vi "测试类型3can请求.vi"(3 "输入切换ID":u8, 4 "输出切换ID":u8) -> (1 "发送成功?":bool)   [LabVIEW 2010]
panel:
  in  "DataLen":i16
  in  "Data":u8[](array[numeric])
  in  "CANPort":u16
  in  "Synchronization":i32(ring)=1 items=["Synchronization"=1, "Asynchronization"=0]
  in  "WriteTimeOut":u32=5000 caption="ms"
  in  "Baudrate":u32(ring)=1000 caption="K" items=["10"=10, "20"=20, "50"=50, "100"=100, "125"=125, "250"=250, "500"=500, "800"=800, "1000"=1000]
  in  "Send_MSG":T1(array[cluster])=[{"Flags"=4, "ID(HEX)"=0, "Data "=[0, 0, 0, 0, 0, 0, 0, 0]}, {"Flags"=4, "ID(HEX)"=0, "Data "=[0, 0, 0, 0, 0, 0, 0, 1]}, {"Flags"=4, "ID(HEX)"=0, "Data "=[0, 0, 0, 0, 0, 0, 0, 2]}, {"Flags"=4, "ID(HEX)"=0, "Data "=[0, 0, 0, 0, 0, 0, 0, 3]}, {"Flags"=4, "ID(HEX)"=0, "Data "=[0, 0, 0, 0, 0, 0, 0, 4]}, {"Flags"=4, "ID(HEX)"=0, "Data "=[0, 0, 0, 0, 0, 0, 0, 5]}, {"Flags"=4, "ID(HEX)"=0, "Data "=[0, 0, 0, 0, 0, 0, 0, 6]}, {"Flags"=4, "ID(HEX)"=0, "Data "=[0, 0, 0, 0, 0, 0, 0, 7]}, {"Flags"=4, "ID(HEX)"=0, "Data "=[0, 0, 0, 0, 0, 0, 0, 8]}, {"Flags"=4, "ID(HEX)"=0, "Data "=[0, 0, 0, 0, 0, 0, 0, 9]}, {"Flags"=4, "ID(HEX)"=0, "Data "=[0, 0, 0, 0, 0, 0, 1, 0]}, {"Flags"=4, "ID(HEX)"=0, "Data "=[0, 0, 0, 0, 0, 0, 1, 1]}, {"Flags"=4, "ID(HEX)"=0, "Data "=[0, 0, 0, 0, 0, 0, 1, 2]}, {"Flags"=4, "ID(HEX)"=0, "Data "=[0, 0, 0, 0, 0, 0, 1, 3]}, {"Flags"=4, "ID(HEX)"=0, "Data "=[0, 0, 0, 0, 0, 0, 1, 4]}, {"Flags"=4, "ID(HEX)"=0, "Data "=[0, 0, 0, 0, 0, 0, 1, 5]}, {"Flags"=4, "ID(HEX)"=0, "Data "=[0, 0, 0, 0, 0, 0, 1, 6]}, {"Flags"=4, "ID(HEX)"=0, "Data "=[0, 0, 0, 0, 0, 0, 1, 7]}, {"Flags"=4, "ID(HEX)"=0, "Data "=[0, 0, 0, 0, 0, 0, 1, 8]}, {"Flags"=4, "ID(HEX)"=0, "Data "=[0, 0, 0, 0, 0, 0, 1, 9]}, {"Flags"=4, "ID(HEX)"=0, "Data "=[0, 0, 0, 0, 0, 0, 2, 0]}, {"Flags"=4, "ID(HEX)"=0, "Data "=[0, 0, 0, 0, 0, 0, 2, 1]}, {"Flags"=4, "ID(HEX)"=0, "Data "=[0, 0, 0, 0, 0, 0, 2, 2]}, {"Flags"=4, "ID(HEX)"=0, "Data "=[0, 0, 0, 0, 0, 0, 2, 3]}, {"Flags"=4, "ID(HEX)"=0, "Data "=[0, 0, 0, 0, 0, 0, 2, 4]}, {"Flags"=4, "ID(HEX)"=0, "Data "=[0, 0, 0, 0, 0, 0, 2, 5]}, {"Flags"=4, "ID(HEX)"=0, "Data "=[0, 0, 0, 0, 0, 0, 2, 6]}, {"Flags"=4, "ID(HEX)"=0, "Data "=[0, 0, 0, 0, 0, 0, 2, 7]}, {"Flags"=4, "ID(HEX)"=0, "Data "=[0, 0, 0, 0, 0, 0, 2, 8]}, {"Flags"=4, "ID(HEX)"=0, "Data "=[0, 0, 0, 0, 0, 0, 2, 9]}, {"Flags"=4, "ID(HEX)"=0, "Data "=[0, 0, 0, 0, 0, 0, 3, 0]}, {"Flags"=4, "ID(HEX)"=0, "Data "=[0, 0, 0, 0, 0, 0, 3, 1]}, {"Flags"=4, "ID(HEX)"=0, "Data "=[0, 0, 0, 0, 0, 0, 3, 2]}, {"Flags"=4, "ID(HEX)"=0, "Data "=[0, 0, 0, 0, 0, 0, 3, 3]}, {"Flags"=4, "ID(HEX)"=0, "Data "=[0, 0, 0, 0, 0, 0, 3, 4]}, {"Flags"=4, "ID(HEX)"=0, "Data "=[0, 0, 0, 0, 0, 0, 3, 5]}, {"Flags"=4, "ID(HEX)"=0, "Data "=[0, 0, 0, 0, 0, 0, 3, 6]}, {"Flags"=4, "ID(HEX)"=0, "Data "=[0, 0, 0, 0, 0, 0, 3, 7]}, {"Flags"=4, "ID(HEX)"=0, "Data "=[0, 0, 0, 0, 0, 0, 3, 8]}, {"Flags"=4, "ID(HEX)"=0, "Data "=[0, 0, 0, 0, 0, 0, 3, 9]}, {"Flags"=4, "ID(HEX)"=0, "Data "=[0, 0, 0, 0, 0, 0, 4, 0]}, {"Flags"=4, "ID(HEX)"=0, "Data "=[0, 0, 0, 0, 0, 0, 4, 1]}, {"Flags"=4, "ID(HEX)"=0, "Data "=[0, 0, 0, 0, 0, 0, 4, 2]}, {"Flags"=4, "ID(HEX)"=0, "Data "=[0, 0, 0, 0, 0, 0, 4, 3]}, {"Flags"=4, "ID(HEX)"=0, "Data "=[0, 0, 0, 0, 0, 0, 4, 4]}, {"Flags"=4, "ID(HEX)"=0, "Data "=[0, 0, 0, 0, 0, 0, 4, 5]}, {"Flags"=4, "ID(HEX)"=0, "Data "=[0, 0, 0, 0, 0, 0, 4, 6]}, {"Flags"=4, "ID(HEX)"=0, "Data "=[0, 0, 0, 0, 0, 0, 4, 7]}, {"Flags"=4, "ID(HEX)"=0, "Data "=[0, 0, 0, 0, 0, 0, 4, 8]}, {"Flags"=4, "ID(HEX)"=0, "Data "=[0, 0, 0, 0, 0, 0, 4, 9]}, {"Flags"=4, "ID(HEX)"=0, "Data "=[0, 0, 0, 0, 0, 0, 5, 0]}, {"Flags"=4, "ID(HEX)"=0, "Data "=[0, 0, 0, 0, 0, 0, 5, 1]}, {"Flags"=4, "ID(HEX)"=0, "Data "=[0, 0, 0, 0, 0, 0, 5, 2]}, {"Flags"=4, "ID(HEX)"=0, "Data "=[0, 0, 0, 0, 0, 0, 5, 3]}, {"Flags"=4, "ID(HEX)"=0, "Data "=[0, 0, 0, 0, 0, 0, 5, 4]}, {"Flags"=4, "ID(HEX)"=0, "Data "=[0, 0, 0, 0, 0, 0, 5, 5]}, {"Flags"=4, "ID(HEX)"=0, "Data "=[0, 0, 0, 0, 0, 0, 5, 6]}, {"Flags"=4, "ID(HEX)"=0, "Data "=[0, 0, 0, 0, 0, 0, 5, 7]}, {"Flags"=4, "ID(HEX)"=0, "Data "=[0, 0, 0, 0, 0, 0, 5, 8]}, {"Flags"=4, "ID(HEX)"=0, "Data "=[0, 0, 0, 0, 0, 0, 5, 9]}, {"Flags"=4, "ID(HEX)"=0, "Data "=[0, 0, 0, 0, 0, 0, 6, 0]}, {"Flags"=4, "ID(HEX)"=0, "Data "=[0, 0, 0, 0, 0, 0, 6, 1]}, {"Flags"=4, "ID(HEX)"=0, "Data "=[0, 0, 0, 0, 0, 0, 6, 2]}, {"Flags"=4, "ID(HEX)"=0, "Data "=[0, 0, 0, 0, 0, 0, 6, 3]}, {"Flags"=4, "ID(HEX)"=0, "Data "=[0, 0, 0, 0, 0, 0, 6, 4]}, {"Flags"=4, "ID(HEX)"=0, "Data "=[0, 0, 0, 0, 0, 0, 6, 5]}, {"Flags"=4, "ID(HEX)"=0, "Data "=[0, 0, 0, 0, 0, 0, 6, 6]}, {"Flags"=4, "ID(HEX)"=0, "Data "=[0, 0, 0, 0, 0, 0, 6, 7]}, {"Flags"=4, "ID(HEX)"=0, "Data "=[0, 0, 0, 0, 0, 0, 6, 8]}, {"Flags"=4, "ID(HEX)"=0, "Data "=[0, 0, 0, 0, 0, 0, 6, 9]}, {"Flags"=4, "ID(HEX)"=0, "Data "=[0, 0, 0, 0, 0, 0, 7, 0]}, {"Flags"=4, "ID(HEX)"=0, "Data "=[0, 0, 0, 0, 0, 0, 7, 1]}, {"Flags"=4, "ID(HEX)"=0, "Data "=[0, 0, 0, 0, 0, 0, 7, 2]}, {"Flags"=4, "ID(HEX)"=0, "Data "=[0, 0, 0, 0, 0, 0, 7, 3]}, {"Flags"=4, "ID(HEX)"=0, "Data "=[0, 0, 0, 0, 0, 0, 7, 4]}, {"Flags"=4, "ID(HEX)"=0, "Data "=[0, 0, 0, 0, 0, 0, 7, 5]}, {"Flags"=4, "ID(HEX)"=0, "Data "=[0, 0, 0, 0, 0, 0, 7, 6]}, {"Flags"=4, "ID(HEX)"=0, "Data "=[0, 0, 0, 0, 0, 0, 7, 7]}, {"Flags"=4, "ID(HEX)"=0, "Data "=[0, 0, 0, 0, 0, 0, 7, 8]}, {"Flags"=4, "ID(HEX)"=0, "Data "=[0, 0, 0, 0, 0, 0, 7, 9]}, {"Flags"=4, "ID(HEX)"=0, "Data "=[0, 0, 0, 0, 0, 0, 8, 0]}, {"Flags"=4, "ID(HEX)"=0, "Data "=[0, 0, 0, 0, 0, 0, 8, 1]}, {"Flags"=4, "ID(HEX)"=0, "Data "=[0, 0, 0, 0, 0, 0, 8, 2]}, {"Flags"=4, "ID(HEX)"=0, "Data "=[0, 0, 0, 0, 0, 0, 8, 3]}, {"Flags"=4, "ID(HEX)"=0, "Data "=[0, 0, 0, 0, 0, 0, 8, 4]}, {"Flags"=4, "ID(HEX)"=0, "Data "=[0, 0, 0, 0, 0, 0, 8, 5]}, {"Flags"=4, "ID(HEX)"=0, "Data "=[0, 0, 0, 0, 0, 0, 8, 6]}, {"Flags"=4, "ID(HEX)"=0, "Data "=[0, 0, 0, 0, 0, 0, 8, 7]}, {"Flags"=4, "ID(HEX)"=0, "Data "=[0, 0, 0, 0, 0, 0, 8, 8]}, {"Flags"=4, "ID(HEX)"=0, "Data "=[0, 0, 0, 0, 0, 0, 8, 9]}, {"Flags"=4, "ID(HEX)"=0, "Data "=[0, 0, 0, 0, 0, 0, 9, 0]}, {"Flags"=4, "ID(HEX)"=0, "Data "=[0, 0, 0, 0, 0, 0, 9, 1]}, {"Flags"=4, "ID(HEX)"=0, "Data "=[0, 0, 0, 0, 0, 0, 9, 2]}, {"Flags"=4, "ID(HEX)"=0, "Data "=[0, 0, 0, 0, 0, 0, 9, 3]}, {"Flags"=4, "ID(HEX)"=0, "Data "=[0, 0, 0, 0, 0, 0, 9, 4]}, {"Flags"=4, "ID(HEX)"=0, "Data "=[0, 0, 0, 0, 0, 0, 9, 5]}, {"Flags"=4, "ID(HEX)"=0, "Data "=[0, 0, 0, 0, 0, 0, 9, 6]}, {"Flags"=4, "ID(HEX)"=0, "Data "=[0, 0, 0, 0, 0, 0, 9, 7]}, {"Flags"=4, "ID(HEX)"=0, "Data "=[0, 0, 0, 0, 0, 0, 9, 8]}, {"Flags"=4, "ID(HEX)"=0, "Data "=[0, 0, 0, 0, 0, 0, 9, 9]}] {"Data" format="%x"; "Flags" items=["MSG_STD"=0, "MSG_EXT"=4]; "ID(HEX)" format="%x"}
  out "Error out":errorcluster {"code" format="%.0x"}
  in  "CANID":u32 format="%x"
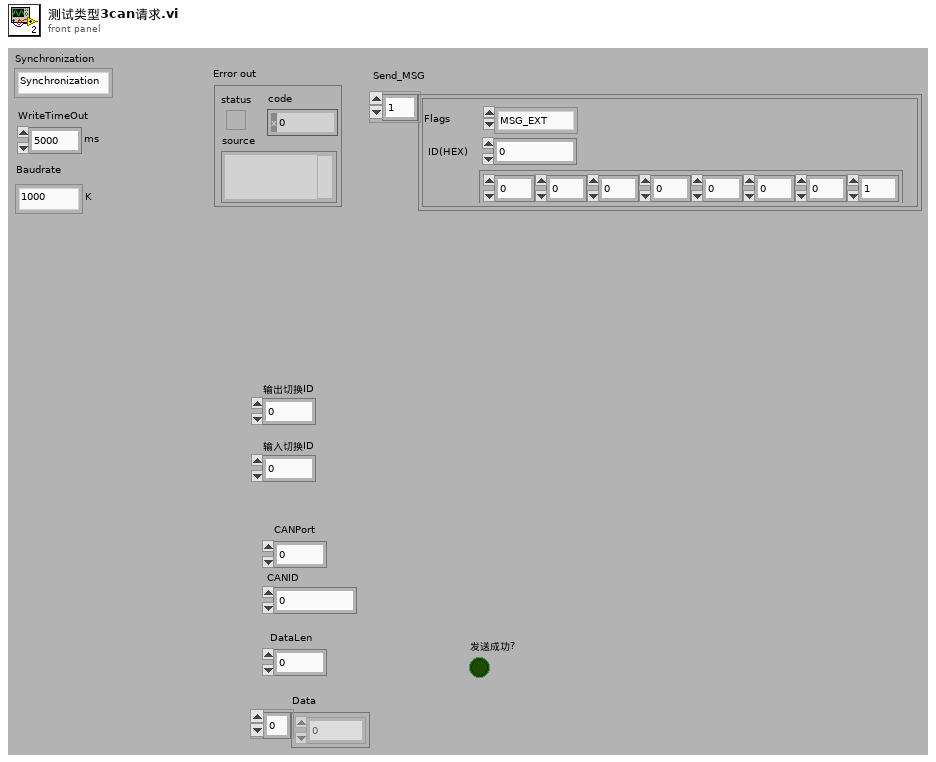
[diagram p1: front panel]
types:
  T1 = cluster{"Flags":u32, "ID(HEX)":u32, "Data ":u8[]}[]
  T2 = cluster{"Internal":u32, "InternalHigh":u32, "Offset":u32, "OffsetHigh":u32, "hEvent":u32}
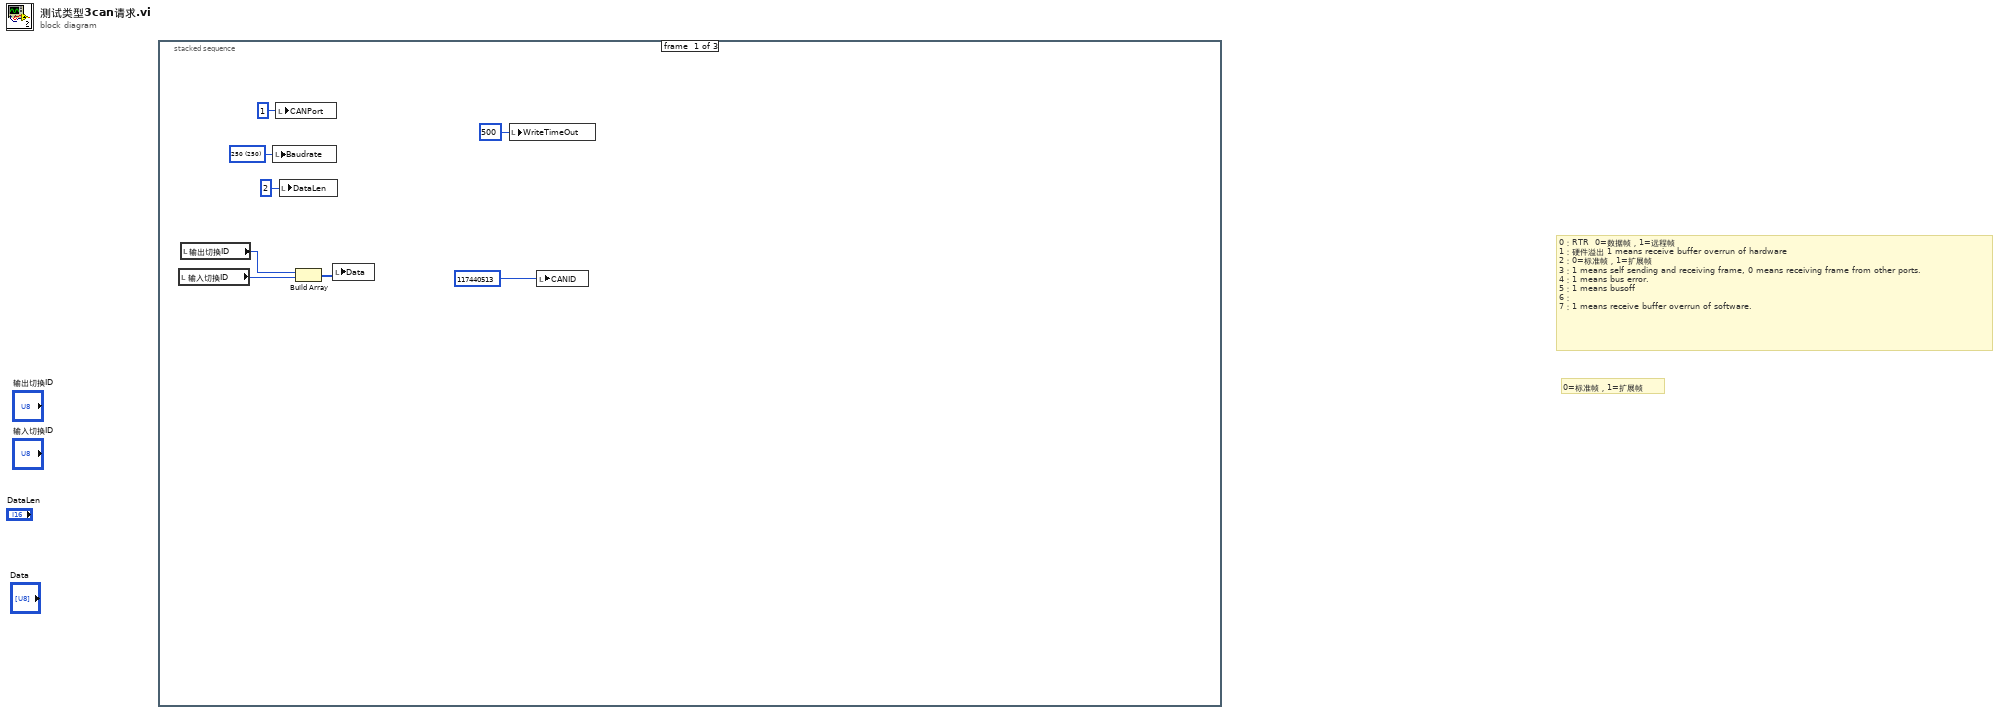
[diagram p0: block diagram]
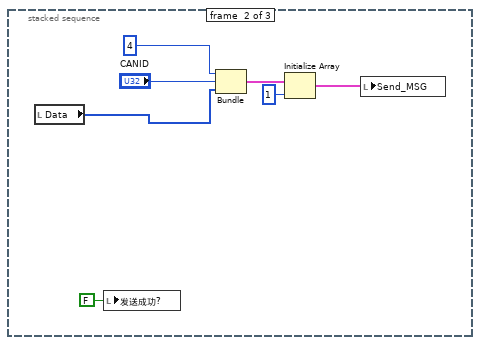
[diagram p2: hidden frame]
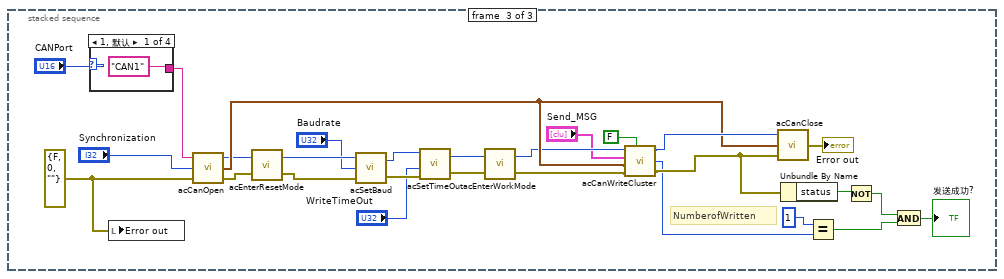
[diagram p3: hidden frame]
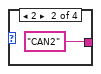
[diagram p4: hidden frame]
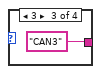
[diagram p5: hidden frame]
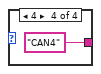
[diagram p6: hidden frame]
diagram:
  # "0=标准帧，1=扩展帧"
  # "0：RTR  0=数据帧，1=远程帧\n1：硬件溢出 1 means receive buffer overrun of hardware\n2：0=标准帧，1=扩展帧\n3：1 means self sending and receiving frame, 0 means receiving frame from other ports.\n4：1 means bus error.\n5：1 means busoff\n6：\n7：1 means receive buffer overrun of software."
  n1 = stacked-sequence {
    frame #0 {
      w8 = u32 250 items=["10"=10, "20"=20, "50"=50, "100"=100, "125"=125, "250"=250, "500"=500, "800"=800, "1000"=1000] ("Baudrate")
      n2 = local read "输入切换ID"() -> (w3:u8)
      n3 = local read "输出切换ID"() -> (w4:u8)
      n4 = local write "Baudrate"(w8) -> ()
      n5 = local write "CANPort"(u16 1 ("CANPort")) -> ()
      n6 = local write "DataLen"(i16 2 ("DataLen")) -> ()
      n7 = Build Array(w4, w3) -> (w5:u8[])
      n8 = local write "Data"(w5) -> ()
      n9 = local write "WriteTimeOut"(u32 500 ("WriteTimeOut")) -> ()
      n10 = local write "CANID"(u32 117440513 ("CANID")) -> ()
    }
    frame #1 {
      n11 = local read "Data"() -> (w9:u8[])
      n12 = local write "发送成功?"(FALSE ("发送成功?")) -> ()
      n13 = Bundle(u32 4, "CANID"="CANID", "Data"=w9) -> (w15:cluster{u32, "CANID":u32, "Data":u8[]})  [unwired: 1 in]
      n14 = Initialize Array(w15, 1 ("维数大小")) -> (w11:cluster{u32, "CANID":u32, "Data":u8[]}[])
      n15 = local write "Send_MSG"(w11) -> ()
    }
    frame #2 {
      w33 = errorcluster {"status"=FALSE, "code"=0, "source"=""} ("Error in")
      # "NumberofWritten"
      n16 = case shown="1, 默认" "CANPort" {
        tunnel: ["CAN1" "CAN2" "CAN3" "CAN4"] -> w25
        frame 1, Default {
        }
        frame 2 {
        }
        frame 3 {
        }
        frame 4 {
        }
      }
      n17 = local write "Error out"(w33) -> ()
      n18 = call "acCanOpen.vi"("Error in"=w33, "Synchronization"="Synchronization", "CANPort"=w25) -> ("Error out"=w30:errorcluster, "Overlapped"=w41:T2, "Handle"=w31:u32)
      n19 = call "acEnterResetMode.vi"("Error in"=w30, "Handle  in"=w31) -> ("Error out"=w39:errorcluster, "Handle out"=w38:u32)
      n20 = call "acSetBaud.vi"("Error in"=w39, "Baudrate"="Baudrate", "Handle  in"=w38) -> ("Error out"=w40:errorcluster, "Handle out"=w27:u32)
      n21 = call "acSetTimeOut.vi"("Error in"=w40, "WriteTimeOut"="WriteTimeOut", "Handle  in"=w27) -> ("Error out"=w34:errorcluster, "Handle out"=w35:u32)  [unwired: 1 in]
      n22 = call "acEnterWorkMode.vi"("Error in"=w34, "Handle  in"=w35) -> ("Error out"=w29:errorcluster, "Handle out"=w28:u32)
      n23 = call "acCanWriteCluster.vi"("Handle  in"=w28, "MSG"="Send_MSG", "Overlapped"=w41, "Error in"=w29, "MSG_RTR"=FALSE) -> ("Handle out"=w42:u32, "NumberOfWritten"=w16:u32, "Error out"=w43:errorcluster)
      n24 = call "acCanClose.vi"("Error in"=w43, "Overlapped"=w41, "Handle  in"=w42) -> ("Error out"=→"Error out":errorcluster)
      n25 = Unbundle By Name(w43) -> ("status"=w21:bool)
      n26 = Equal?(x=u32 1, y=w16) -> (x = y?=w19:bool)
      n27 = Not(x=w21) -> (.not. x?=w22:bool)
      n28 = And(x=w22, y=w19) -> (x .and. y?=→"发送成功?":bool)
    }
  }
